vi "axex_close_file_office16.vi"(5 "close file in Excel (False)":bool, 6 "file overwrite prompt (True)":bool=TRUE, 7 "force operation (ingnore error in) (True)":bool=TRUE, 8 "error in":errorcluster, 9 "save path (no path)":path, 10 "save changes (True)":bool=TRUE, 11 "AX Excel instance in":T1) -> (0 "error out":errorcluster)   [LabVIEW 2020, in "AX Excel.lvlib"]
doc: "Note: Office 2016 version - disabled SaveAs() method, excel file must be opened, not created!\n\nCall this to close given excel file. 'save changes?' option saves changes in the file. 'close file' option will close the file in M$ Excel application. If current workbook is new workbook (not loaded from file) or you want to change file destination you can optionally specify save path. If it is new workbook and no path is given the save dialog will be displayed.\nThis VI optionally ignores errors so it will try to save even if there is some error in error wire."
uses:
  AX Excel.lvlib
  axex_instance.ctl
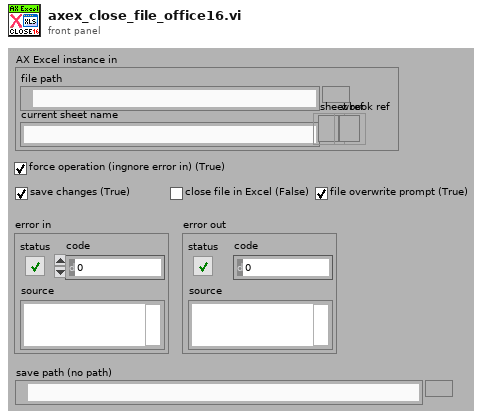
[diagram p1: front panel]
types:
  T1 = typedef "AX Excel.lvlib/axex_instance.ctl" = cluster{"file path":path, "current sheet name":string, "sheet ref":refnum<k7>, "wbook ref":refnum<k7>}
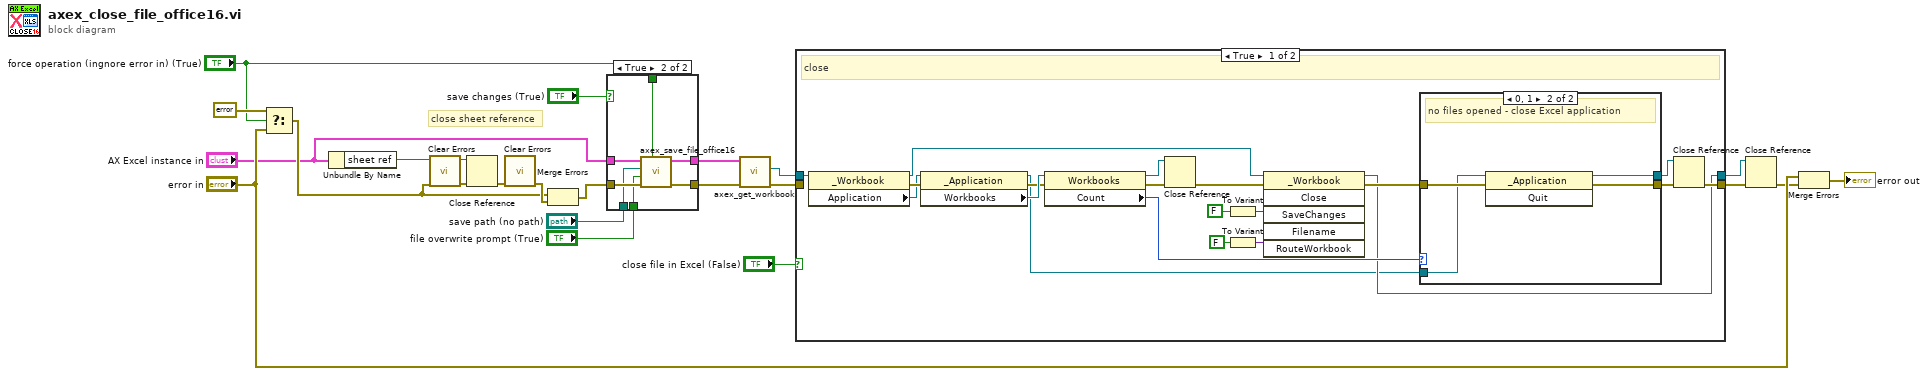
[diagram p0: block diagram]
diagram:
  # "close sheet reference"
  n1 = Select(t=errorcluster {"status"=FALSE, "code"=0, "source"=""}, s="force operation (ingnore error in) (True)", f="error in") -> (s? t:f=w14:errorcluster)
  n2 = Unbundle By Name("AX Excel instance in") -> ("sheet ref"=w18:refnum<k7>)
  n3 = call <vilib>:"Clear Errors.vi"("error in (no error)"=w14) -> ("error out"=w16:errorcluster)  [unwired: 5 in, 1 out]
  n4 = Close Reference(reference=w18, error in (no error)=w16) -> (error out=w17:errorcluster)
  n5 = call <vilib>:"Clear Errors.vi"("error in (no error)"=w17) -> ("error out"=w15:errorcluster)  [unwired: 5 in, 1 out]
  n6 = Merge Errors(w14, w15) -> (w8:errorcluster)
  n7 = case shown="True" "save changes (True)" {
    tunnel: [w24 w31] -> w9
    tunnel: w8 -> [w24 w30]
    tunnel: [w23 w29] -> w7
    tunnel: "AX Excel instance in" -> [w23 w28]
    tunnel: "save path (no path)" -> [_ w27]
    tunnel: "force operation (ingnore error in) (True)" -> [_ w26]
    tunnel: "file overwrite prompt (True)" -> [_ w25]
    frame False {
    }
    frame True {
      n8 = call "axex_save_file_office16.vi"("force operation (ignore error in) (True)"=w26, "error in"=w30, "file overwrite prompt (True)"=w25, "file path (no path)"=w27, "AX Excel instance in"=w28) -> ("error out"=w31:errorcluster, "AX Excel instance out"=w29:T1)  [unwired: 5 in]
    }
  }
  n9 = call "axex_get_workbook.vi"("error in"=w9, "AX Excel instance in"=w7) -> ("error out"=w2:errorcluster, "excel workbook"=w19:refnum<k7>)  [unwired: 7 in, 1 out]
  n10 = case shown="True" "close file in Excel (False)" {
    tunnel: w19 -> [w45 w58]
    tunnel: [w47 w59] -> w13
    tunnel: [w38 w58] -> w11
    tunnel: w2 -> [_ w59]
    frame True {
      # "close"
      n11 = property class="_Workbook"(reference=w45) -> (reference out=w39:refnum<k7>, error out=w37:errorcluster, "Application"=w36:refnum<k7>)  [unwired: 1 in]
      n12 = property class="_Application"(reference=w36, error in=w37) -> (reference out=w33:refnum<k7>, error out=w34:errorcluster, "Workbooks"=w35:refnum<k7>)
      n13 = property class="Workbooks"(reference=w35, error in=w34) -> (reference out=w50:refnum<k7>, error out=w51:errorcluster, "Count"=w49:i32)
      n14 = Close Reference(reference=w50, error in (no error)=w51) -> (error out=w41:errorcluster)
      n15 = To Variant(anything=FALSE) -> (Variant=w44:variant)
      n16 = To Variant(anything=FALSE) -> (Variant=w43:variant)
      n17 = invoke class="_Workbook" method="Close"(reference=w39, error in=w41, "SaveChanges"=w44, "RouteWorkbook"=w43) -> (reference out=w38:refnum<k7>, error out=w40:errorcluster)  [unwired: 2 in, 4 out]
      n18 = case shown="0, 1" w49 {
        tunnel: w40 -> [w53 w57]
        tunnel: w33 -> [w52 w56]
        tunnel: [w53 w55] -> w48
        tunnel: [w52 w54] -> w46
        frame Default {
          # "some more files opened - let Excel running"
        }
        frame 0, 1 {
          # "no files opened - close Excel application"
          n19 = invoke class="_Application" method="Quit"(reference=w56, error in=w57) -> (reference out=w54:refnum<k7>, error out=w55:errorcluster)  [unwired: 1 in, 1 out]
        }
      }
      n20 = Close Reference(reference=w46, error in (no error)=w48) -> (error out=w47:errorcluster)
    }
    frame False {
      # "save only"
    }
  }
  n21 = Close Reference(reference=w11, error in (no error)=w13) -> (error out=w12:errorcluster)
  n22 = Merge Errors("error in", w12) -> (→"error out":errorcluster)
